vi "SRV_Main Config Paths.vi"(0 "local data":T1 {"Motor Control Config"."Release Cmds"."Motor Control Commands Array"."Value" format="%02x"; "Motor Control Config"."Release Cmds"."Motor Control Commands Array"."Register" format="%02x"; "Motor Control Config"."Release Cmds"."Motor Control Commands Array"."I2C Address" format="%02x"; "Motor Control Config"."Press Cmds"."Motor Control Commands Array"."Value" format="%02x"; "Motor Control Config"."Press Cmds"."Motor Control Commands Array"."Register" format="%02x"; "Motor Control Config"."Press Cmds"."Motor Control Commands Array"."I2C Address" format="%02x"}) -> (4 "local data dup":T1 {"Motor Control Config"."Release Cmds"."Motor Control Commands Array"."Value" format="%02x"; "Motor Control Config"."Release Cmds"."Motor Control Commands Array"."Register" format="%02x"; "Motor Control Config"."Release Cmds"."Motor Control Commands Array"."I2C Address" format="%02x"; "Motor Control Config"."Press Cmds"."Motor Control Commands Array"."Value" format="%02x"; "Motor Control Config"."Press Cmds"."Motor Control Commands Array"."Register" format="%02x"; "Motor Control Config"."Press Cmds"."Motor Control Commands Array"."I2C Address" format="%02x"}, 6 "SystemConfig Filepath":path, 8 "MotorsConfig Filepath":path, 10 "SensorsConfig Filepath":path, 12 "SensorsConfig regexp":string, 13 "MotorsConfig regexp":string, 14 "SystemConfig regexp":string)   [LabVIEW 2009]
uses:
  SRV_Main Controller Local Data.ctl
  Motors/Motors Config/SRV_Motor Control Button Config.ctl
  Motors/Motors Config/SRV_Motor Legos-Servo.ctl
  Motors/Motors Config/SRV_Motor Control Commands Cluster.ctl
  Motors/Motors Config/SRV_Motor Control Command Config.ctl
  Motors/Motors Config/SRV_Motor Control Button Icons_FALSE.ctl
  SubVIs/SRV_Streaming States.ctl
  SubVIs/SRV_Streaming State.ctl
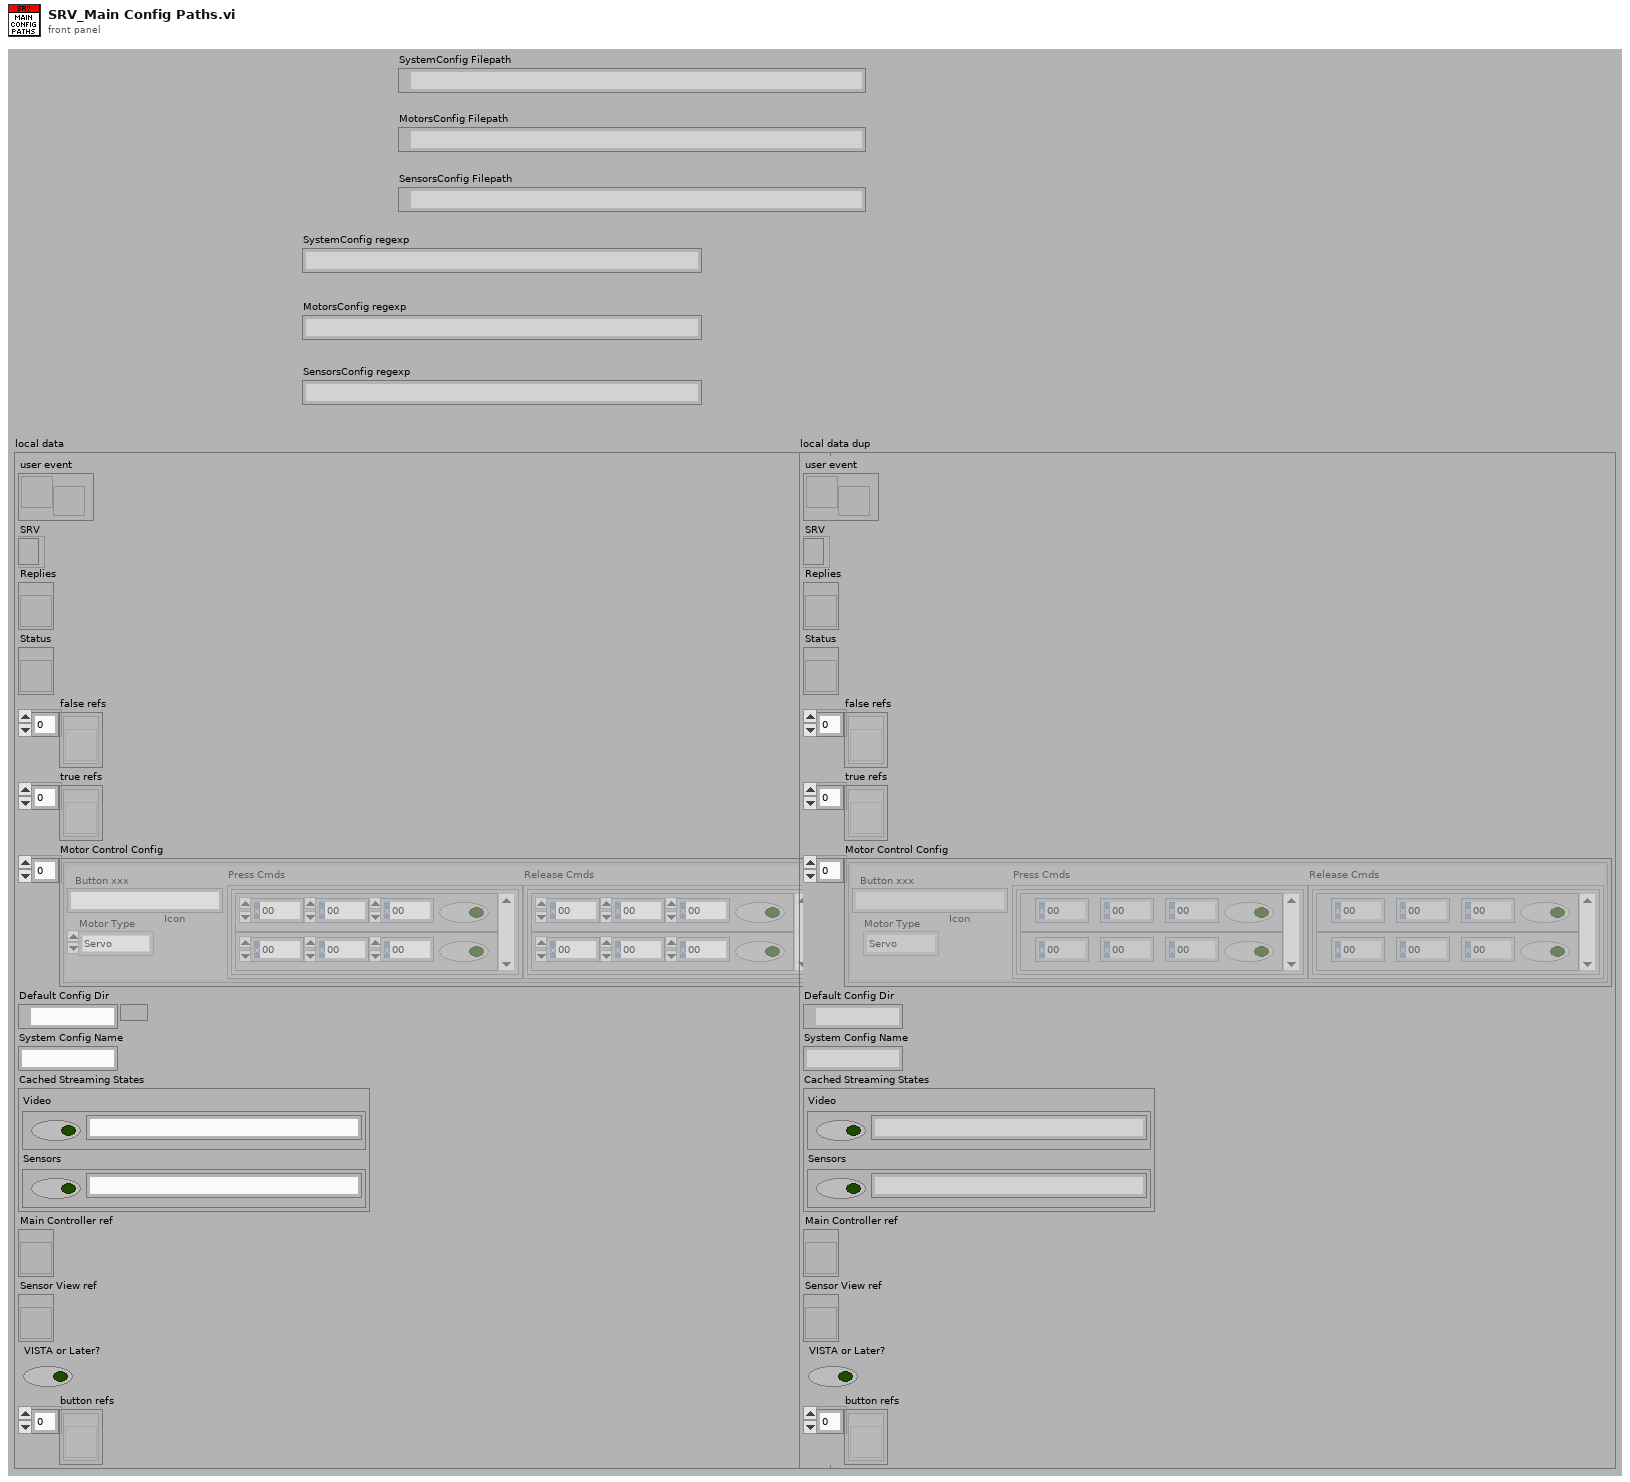
[diagram p1: front panel]
types:
  T1 = typedef "SRV_Main Controller Local Data.ctl" = cluster{"user event":refnum<user-event>, "SRV":refnum<k5>, "Replies":refnum<vi>, "Status":refnum<vi>, "false refs":refnum<vi>[], "true refs":refnum<vi>[], "Motor Control Config":T2[], "Default Config Dir":path, "System Config Name":string, "Cached Streaming States":T7, "Main Controller ref":refnum<vi>, "Sensor View ref":refnum<vi>, "VISTA or Later?":bool, "button refs":refnum<vi>[]}
  T2 = typedef "SRV_Motor Control Button Config.ctl" = cluster{"Button Name":string, "Button Label":string, "Motor Type":T3, "Press Cmds":T4, "Release Cmds":T4, "Icon":T6}
  T3 = typedef "SRV_Motor Legos-Servo.ctl" = enum16{"Servo", "Legos", "Shared Var"}
  T4 = typedef "SRV_Motor Control Commands Cluster.ctl" = cluster{"Motor Control Commands Array":T5[]}
  T5 = typedef "SRV_Motor Control Command Config.ctl" = cluster{"I2C Address":u8, "Register":u8, "Value":u8, "Active":bool}
  T6 = typedef "SRV_Motor Control Button Icons_FALSE.ctl" = u16
  T7 = typedef "SRV_Streaming States.ctl" = cluster{"Video":T8, "Sensors":T8}
  T8 = typedef "SRV_Streaming State.ctl" = cluster{"Enabled":bool, "Data":string}
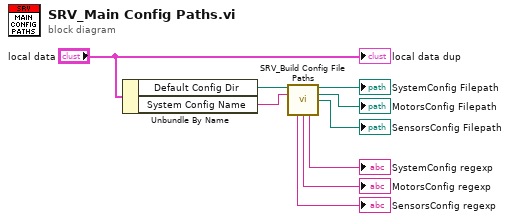
[diagram p0: block diagram]
diagram:
  n1 = Unbundle By Name("local data") -> ("Default Config Dir"=w9:path, "System Config Name"=w8:string)
  n2 = call "SRV_Build Config File Paths.vi"("Config Dir"=w9, "Sys Config Name"=w8) -> ("SystemConfig Filepath"=→"SystemConfig Filepath":path, "MotorsConfig Filepath"=→"MotorsConfig Filepath":path, "SensorsConfig Filepath"=→"SensorsConfig Filepath":path, "SensorsConfig regexp"=→"SensorsConfig regexp":string, "MotorsConfig regexp"=→"MotorsConfig regexp":string, "SystemConfig regexp"=→"SystemConfig regexp":string)  [unwired: 8 in]
  "local data dup" <- "local data"
